vi "Configure Channel Preprocessing.vi"(0 "VISA resource name":refnum<visa-resource-name>, 1 "Update (0: All Properties)":T1(ring), 5 "Channel (0: Channel 1)":u16(ring) items=["Channel 1", "Channel 2", "Channel 3", "Channel 4"], 7 "Interpolation (0: Linear)":u16(ring) items=["Linear", "Sinx/x"], 9 "Noise Filter (0: None)":u16(ring) items=["None", "+0.5 bit", "+1 bit", "+1.5 bits", "+2 bits", "+2.5 bits", "+3 bits"], 11 "error in (no error)":errorcluster, 12 "Sweeps to Average (1)":i32=1 min=1, 13 "Invert (False)":bool) -> (4 "VISA resource name out":refnum<visa-resource-name>, 15 "error out":errorcluster)   [LabVIEW 2013, in "LeCroy Wave Series.lvlib"]
doc: "Controls the Channel Preprocessing features of LeCroy XStream Oscilloscopes."
uses:
  LeCroy Wave Series.lvlib
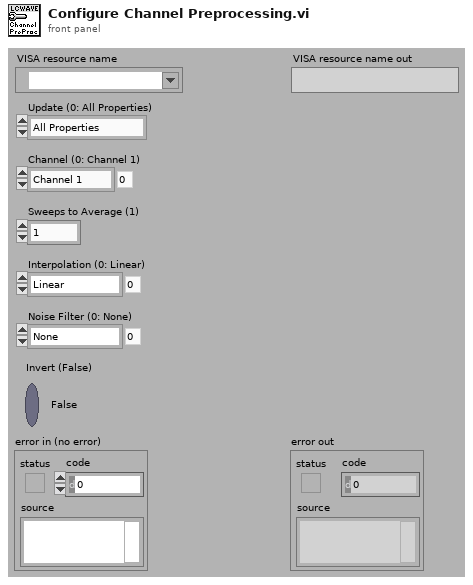
[diagram p1: front panel]
types:
  T1 = enum16{"All Properties", "Averaging", "Interpolation", "Noise Filter", "Invert"}
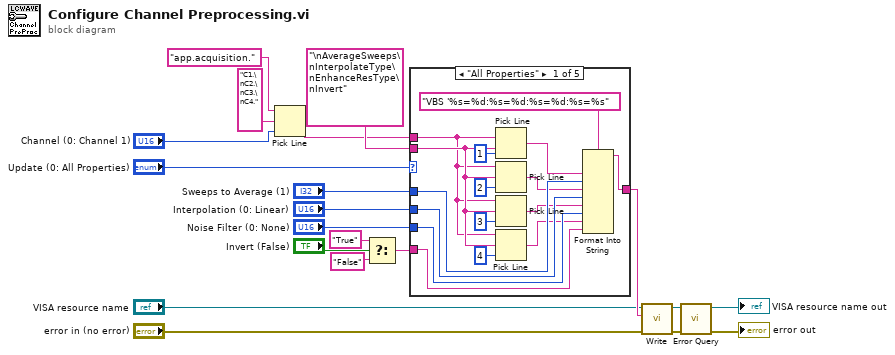
[diagram p0: block diagram]
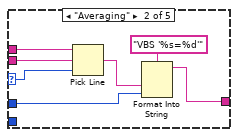
[diagram p2: hidden frame]
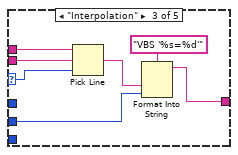
[diagram p3: hidden frame]
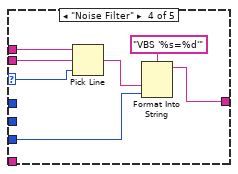
[diagram p4: hidden frame]
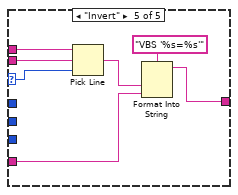
[diagram p5: hidden frame]
diagram:
  n1 = Pick Line(string ("")="app.acquisition." ("format string"), multi-line string="C1.\nC2.\nC3.\nC4.", line index="Channel (0: Channel 1)") -> (output string=w9:string)
  n2 = Select(t="True" ("output string"), s="Invert (False)", f="False" ("output string")) -> (s? t:f=w5:string)
  n3 = case shown="\"All Properties\"" "Update (0: All Properties)" {
    selector: "Update (0: All Properties)" -> [_ w39 w45 w52 w59]
    tunnel: "\nAverageSweeps\nInterpolateType\nEnhanceResType\nInvert" -> [w34 w38 w46 w53 w60]
    tunnel: "Sweeps to Average (1)" -> [w28 w43 _ _ _]
    tunnel: [w35 w41 w49 w56 w63] -> w13
    tunnel: "Interpolation (0: Linear)" -> [w26 _ w48 _ _]
    tunnel: "Noise Filter (0: None)" -> [w25 _ _ w55 _]
    tunnel: w5 -> [w24 _ _ _ w62]
    tunnel: w9 -> [w21 w37 w47 w54 w61]
    frame "All Properties" {
      n4 = Pick Line(string ("")=w21, multi-line string=w34, line index=1) -> (output string=w29:string)
      n5 = Pick Line(string ("")=w21, multi-line string=w34, line index=2) -> (output string=w27:string)
      n6 = Pick Line(string ("")=w21, multi-line string=w34, line index=3) -> (output string=w23:string)
      n7 = Pick Line(string ("")=w21, multi-line string=w34, line index=4) -> (output string=w22:string)
      n8 = Format Into String(format string="VBS '%s=%d:%s=%d:%s=%d:%s=%s", w29, w28, w27, w26, w23, w25, w22, w24) -> (resulting string=w35:string)  [unwired: 2 in, 1 out]
    }
    frame "Averaging" {
      n9 = Pick Line(string ("")=w37, multi-line string=w38, line index=w39) -> (output string=w40:string)
      n10 = Format Into String(format string="VBS '%s=%d'", w40, w43) -> (resulting string=w41:string)  [unwired: 2 in, 1 out]
    }
    frame "Interpolation" {
      n11 = Pick Line(string ("")=w47, multi-line string=w46, line index=w45) -> (output string=w44:string)
      n12 = Format Into String(format string="VBS '%s=%d'", w44, w48) -> (resulting string=w49:string)  [unwired: 2 in, 1 out]
    }
    frame "Noise Filter" {
      n13 = Pick Line(string ("")=w54, multi-line string=w53, line index=w52) -> (output string=w51:string)
      n14 = Format Into String(format string="VBS '%s=%d'", w51, w55) -> (resulting string=w56:string)  [unwired: 2 in, 1 out]
    }
    frame "Invert" {
      n15 = Pick Line(string ("")=w61, multi-line string=w60, line index=w59) -> (output string=w58:string)
      n16 = Format Into String(format string="VBS '%s=%s'", w58, w62) -> (resulting string=w63:string)  [unwired: 2 in, 1 out]
    }
  }
  n17 = call "Write.vi"("error in (no error)"="error in (no error)", "Write Buffer"=w13, "VISA resource name"="VISA resource name") -> ("error out"=w3:errorcluster, "VISA resource name out"=w4:refnum<visa-resource-name>)  [unwired: 6 in, 1 out]
  n18 = call "Error Query.vi"("error in (no error)"=w3, "VISA resource name"=w4) -> ("error out"=→"error out":errorcluster, "VISA resource name out"=→"VISA resource name out":refnum<visa-resource-name>)  [unwired: 6 in, 2 out]
